vi "Get Type.vi"(8 "error in (no error)":errorcluster, 11 "Wood in":refnum<class "Wood.lvclass">) -> (0 "error out":errorcluster, 2 "Item Type":T1, 3 "Wood out":refnum<class "Wood.lvclass">)   [LabVIEW 2020, in "Wood.lvclass"]
uses:
  Wood.lvclass
  Item/Item Type.ctl
  Item/Item.lvclass
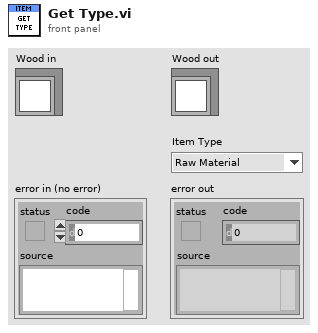
[diagram p1: front panel]
types:
  T1 = typedef "Item.lvclass/Item Type.ctl" = enum16{"Raw Material", "Component", "Module", "Product"}
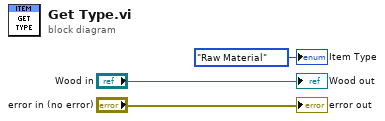
[diagram p0: block diagram]
diagram:
  "error out" <- "error in (no error)"
  "Wood out" <- "Wood in"
  "Item Type" <- Item_Type."Raw Material" ("Item Type")
